vi "meas_cycle_TD_FFT.vi"(2 "PSG freq offset":dbl=0.0003 caption="freq. offset (Hz)" min=0.00025 max=67.0 step=1e-06 format="%#.12p", 3 "time domain array":dbl[](array[numeric]), 4 "dt":dbl, 5 "current frequency":dbl) -> (0 "output time domain signal":waveform(dbl), 1 "output spectrum":T1)   [LabVIEW 2011]
doc: "converts the time domain data to freq. domain data and corrects the frequency offset. \n\nFurthermore, the DC component is deleted from the freq. domain signal."
uses:
  <vilib>/express/express analysis/Spectral/Block/exnSpectralBlock spectral measurements power poly.vi
  <vilib>/express/express analysis/Spectral/Block/exnSpectralBlock spectral measurements power WFM.vi
  <vilib>/express/express analysis/Spectral/XNode/ExpressSpectralMeasurementsBlockNode.xnode
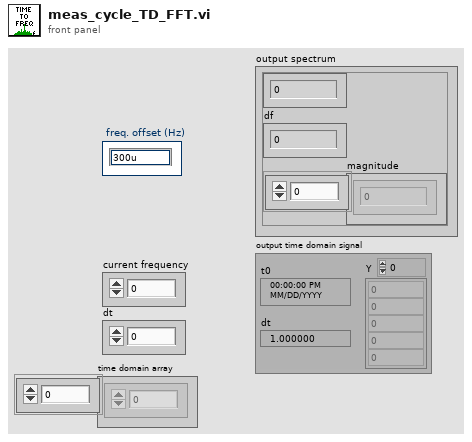
[diagram p1: front panel]
types:
  T1 = cluster{"Numeric Control":dbl, "df":dbl, "magnitude":dbl[]}
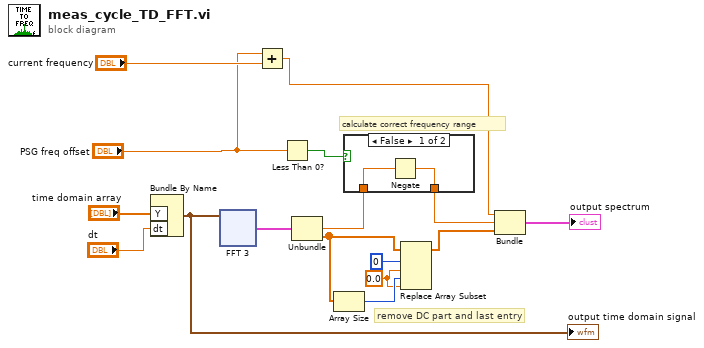
[diagram p0: block diagram]
diagram:
  w9 = 0.0 ("new element/subarray")
  # "calculate correct frequency range"
  # "remove DC part and last entry"
  n1 = Bundle By Name("Y"="time domain array", "dt"="dt") -> (w14:waveform(dbl))  [unwired: 1 in]
  "output time domain signal" <- w14
  n2 = xnode ("FFT 3")("Signals"=w14) -> ("Power Spectrum"=w15:cluster{"f0":dbl, "df":dbl, "magnitude":dbl[]})  [unwired: 1 in, 1 out]
  n3 = Add(x="PSG freq offset", y="current frequency") -> (x+y=w1:dbl)
  n4 = Less Than 0?(x="PSG freq offset") -> (x < 0?=w4:bool)
  n5 = Unbundle(w15) -> ("df"=w6:dbl, "magnitude"=w11:dbl[])  [unwired: 1 out]
  n6 = Array Size(array=w11) -> (size(s)=w10:i32)
  n7 = case shown="False" w4 {
    tunnel: w6 -> [w18 w19]
    tunnel: [w17 w19] -> w5
    frame False {
      n8 = Negate(x=w18) -> (-x=w17:dbl)
    }
    frame True {
    }
  }
  n9 = Replace Array Subset(array=w11, new element #1=w9, index #1=0 ("index"), new element #2=w9, index #2=w10) -> (w8:dbl[])
  n10 = Bundle(w1, "df"=w5, "magnitude"=w8) -> (→"output spectrum":cluster{dbl, "df":dbl, "magnitude":dbl[]})  [unwired: 1 in]
